vi "Unit7.vi"() -> ()   [LabVIEW 2023]
panel:
  in  "Ro - CH3BO3":bool
  in  "Stop":bool
  in  "Графики":bool
  in  "ОРСУЗ":bool
  in  "Реактивност":bool
  in  "Борна концентрация":bool
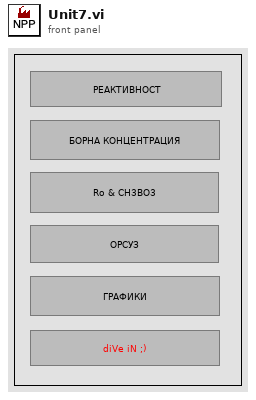
[diagram p1: front panel]
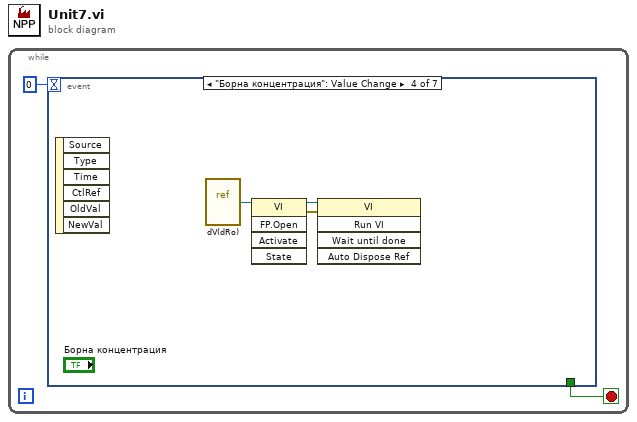
[diagram p0: block diagram]
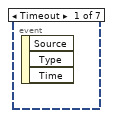
[diagram p2: hidden frame]
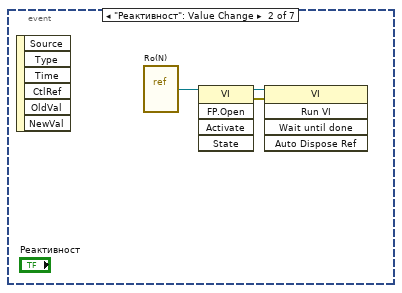
[diagram p3: hidden frame]
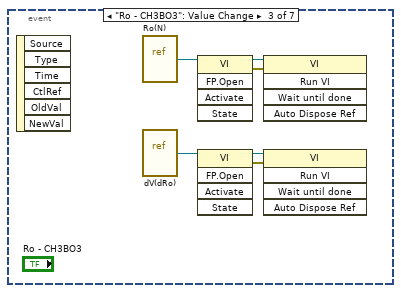
[diagram p4: hidden frame]
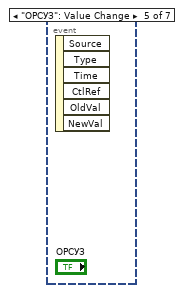
[diagram p5: hidden frame]
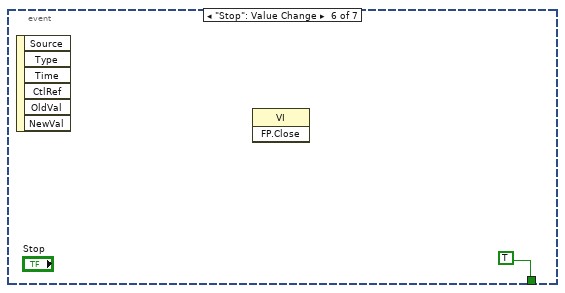
[diagram p6: hidden frame]
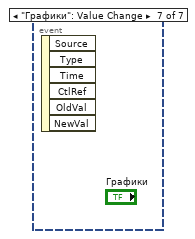
[diagram p7: hidden frame]
diagram:
  n1 = while {
    stop <- w2 stop-if-true
    n2 = event shown="[3] \"Борна концентрация\": Value Change" {
      selector: _ -> [_ _ _ _ _ _ _]
      dyn-events: _ -> [_ _ _ _ _ _ _]
      timeout: 0 -> [_ _ _ _ _ _ _]
      tunnel: [_ _ _ _ _ TRUE _] -> w2
      event Timeout {
        n3 = event-data() -> ()  [unwired: 1 in, 3 out]
      }
      event "Реактивност": Value Change {
        n4 = event-data() -> ()  [unwired: 1 in, 6 out]
        n5 = vi-ref "Ro(N).vi"() -> (w5:refnum<vi>)
        n6 = invoke class="VI" method="FP.Open"(reference=w5) -> (reference out=w4:refnum<vi>, error out=w3:errorcluster)  [unwired: 4 in, 3 out]
        n7 = invoke class="VI" method="Run VI"(reference=w4, error in=w3) -> ()  [unwired: 3 in, 5 out]
      }
      event "Ro - CH3BO3": Value Change {
        n8 = event-data() -> ()  [unwired: 1 in, 6 out]
        n9 = vi-ref "Ro(N).vi"() -> (w11:refnum<vi>)
        n10 = vi-ref "dV(dRo).vi"() -> (w8:refnum<vi>)
        n11 = invoke class="VI" method="FP.Open"(reference=w11) -> (reference out=w10:refnum<vi>, error out=w9:errorcluster)  [unwired: 4 in, 3 out]
        n12 = invoke class="VI" method="FP.Open"(reference=w8) -> (reference out=w7:refnum<vi>, error out=w6:errorcluster)  [unwired: 4 in, 3 out]
        n13 = invoke class="VI" method="Run VI"(reference=w10, error in=w9) -> ()  [unwired: 3 in, 5 out]
        n14 = invoke class="VI" method="Run VI"(reference=w7, error in=w6) -> ()  [unwired: 3 in, 5 out]
      }
      event "Борна концентрация": Value Change {
        n15 = event-data() -> ()  [unwired: 1 in, 6 out]
        n16 = vi-ref "dV(dRo).vi"() -> (w14:refnum<vi>)
        n17 = invoke class="VI" method="FP.Open"(reference=w14) -> (reference out=w13:refnum<vi>, error out=w12:errorcluster)  [unwired: 4 in, 3 out]
        n18 = invoke class="VI" method="Run VI"(reference=w13, error in=w12) -> ()  [unwired: 3 in, 5 out]
      }
      event "ОРСУЗ": Value Change {
        n19 = event-data() -> ()  [unwired: 1 in, 6 out]
      }
      event "Stop": Value Change {
        n20 = event-data() -> ()  [unwired: 1 in, 6 out]
        n21 = invoke class="VI" method="FP.Close"() -> ()  [unwired: 3 in, 3 out]
      }
      event "Графики": Value Change {
        n22 = event-data() -> ()  [unwired: 1 in, 6 out]
      }
    }
  }
